vi "aes_IsAngleCycle.vi"(1 "Crank or Cyle Angle":fxp<+,61,10> format="%.55g") -> (0 "Boolean":bool)   [LabVIEW 2010, in "AES.lvlib" / "AES FPGA.lvlib"]
uses:
  AES FPGA.lvlib
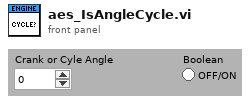
[diagram p1: front panel]
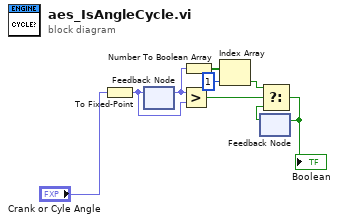
[diagram p0: block diagram]
diagram:
  n1 = To Fixed-Point(number="Crank or Cyle Angle") -> (fixed-point=w2:fxp<+,2,10>)  [unwired: 1 in]
  n2 = feedback #1() -> (w4:fxp<+,2,10>)  [unwired: 1 in]
  n3 = feedback-in #1(w2) -> ()
  n4 = Greater?(x=w4, y=w2) -> (0:w3:bool)
  n5 = Number To Boolean Array(number=w4) -> (Boolean array=w5:bool[])
  n6 = Index Array(array=w5, index=1) -> (element=w7:bool)
  n7 = feedback #2() -> (w8:bool)  [unwired: 1 in]
  n8 = Select(t=w7, s=w3, f=w8) -> (s? t:f=w9:bool)
  "Boolean" <- w9
  n9 = feedback-in #2(w9) -> ()
